vi "movement(a side) fwd use navX and Sonic.vi"(7 "angle Z(align)":ext, 8 "error in (no error)":errorcluster, 11 "distance":dbl) -> (0 "error out":errorcluster, 3 "angle Z":ext)   [LabVIEW 2017]
uses:
  <vilib>/myRIO/Common/Instrument Driver Framework/Utilities/typedefs/Generic FPGA Reference.ctl
  <vilib>/myRIO/Common/Instrument Driver Framework/Utilities/typedefs/myRIO v1.0 Reference.ctl
  <vilib>/myRIO/Common/Instrument Driver Framework/Utilities/typedefs/Hardware Version Enum.ctl
  <vilib>/myRIO/Common/Instrument Driver Framework/Utilities/typedefs/myRIO Generic Hardware Reference.ctl
  <vilib>/Instr/_visa.llb/VISA Configure Serial Port (Instr).vi
  <vilib>/userdefined/High Color/nirio_resource_hc.ctl
  <vilib>/myRIO/Common/Instrument Driver Framework/myRIO v1.0/Encoder/typedefs/Encoder Count Direction Enum.ctl
  <vilib>/myRIO/Common/Instrument Driver Framework/myRIO v1.0/Encoder/typedefs/Encoder Signal Mode.ctl
  <vilib>/myRIO/Common/Instrument Driver Framework/myRIO v1.0/Encoder/typedefs/Encoder Channels Enum.ctl
  <vilib>/myRIO/Instrument Drivers/Onboard IO/Encoder/typedefs/Encoder Reference.ctl
  <vilib>/myRIO/Instrument Drivers/Onboard IO/Encoder/Encoder.lvlib
  <vilib>/myRIO/Instrument Drivers/Onboard IO/Encoder/vis/Read.vi
  <vilib>/myRIO/Common/Instrument Driver Framework/myRIO v1.0/Encoder/typedefs/Encoder Configuration v1.0.ctl
  <vilib>/myRIO/Common/Instrument Driver Framework/myRIO v1.0/Encoder/vis/myRIO v1.1 Open Encoder.vi
  <vilib>/myRIO/Common/Instrument Driver Framework/myRIO v1.0/Encoder/vis/myRIO v1.0 Configure Encoder.vi
  <vilib>/myRIO/Instrument Drivers/Onboard IO/Encoder/vis/myRIO Encoder Open.xnode
  <vilib>/myRIO/Common/Instrument Driver Framework/Utilities/vis/Is FPGA Ref Available.vi
  <vilib>/myRIO/Express VI/Onboard IO/Encoder/Encoder Express VI.xnode
  <vilib>/myRIO/Instrument Drivers/Onboard IO/I2C/typedefs/I2C Transfer Rate.ctl
  <vilib>/myRIO/Instrument Drivers/Onboard IO/I2C/I2C.lvlib
  <vilib>/myRIO/Instrument Drivers/Onboard IO/I2C/typedefs/I2C Configuration.ctl
  <vilib>/myRIO/Common/Instrument Driver Framework/myRIO v1.0/I2C/typedefs/I2C Channels Enum.ctl
  <vilib>/myRIO/Instrument Drivers/Onboard IO/I2C/typedefs/I2C Reference.ctl
  <vilib>/myRIO/Instrument Drivers/Onboard IO/I2C/vis/myRIO I2C Open.xnode
  <vilib>/myRIO/Instrument Drivers/Utilities/Utilities.lvlib
  <vilib>/imath/engines/lvmath2/RunTimeEngine/Managers/WorkSpace/UID Generator.vi
  <vilib>/imath/engines/lvmath2/RunTimeEngine/LocalVariableDefStatement/MC_LocalVariableDefStatement_Display.vi
  <vilib>/imath/engines/lvmath2/RunTimeEngine/RunTimeType/NIMS_RunTimeType_From StrictType (excl LVString).vi
  <vilib>/imath/engines/lvmath2/RunTimeEngine/Managers/SymbolTable/Clear UID.vi
  <vilib>/imath/engines/lvmath2/RunTimeEngine/Managers/SymbolTable/NIMS_WorkSpace.lvlib
  <vilib>/imath/engines/lvmath2/RunTimeEngine/NodeEndStatement/NIMS_NodeEndStatement_Output.vi
  <vilib>/imath/engines/lvmath2/RunTimeEngine/ErrorHandling/NIMS_Finalize Error.vi
  <vilib>/imath/engines/lvmath2/RunTimeEngine/BuiltInFunctions/abs/NIMS_abs(signed).vi
  <vilib>/myRIO/Common/Instrument Driver Framework/myRIO v1.0/I2C/vis/myRIO v1.1 Open I2C.vi
panel:
  out "value Z":ext
  out "left_pwm":dbl
  out "right_pwm":dbl
  in  "stop":bool
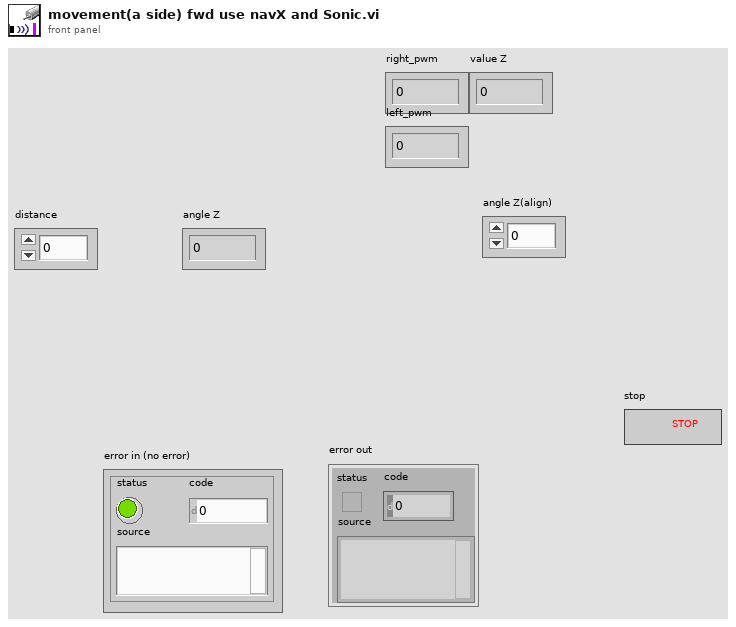
[diagram p1: front panel]
types:
  T1 = typedef "I2C.lvlib/I2C Reference.ctl" = cluster{"myRIO Reference":T2, "I2C Channels Enum":T6, "I2C Configuration":T7}
  T2 = typedef "myRIO Generic Hardware Reference.ctl" = cluster{"myRIO Model":T3, "myRIO Hardware Reference":T4}
  T3 = typedef "Hardware Version Enum.ctl" = enum16{"Unknown", "myRIO-1900", "myRIO-1950", "roboRIO", "NI ELVIS RIO CM"}
  T4 = typedef "myRIO v1.0 Reference.ctl" = cluster{"Generic FPGA Reference":T5, "Allow multiple opens":bool}
  T5 = typedef "Generic FPGA Reference.ctl" = refnum<k20>
  T6 = typedef "I2C Channels Enum.ctl" = enum16{"Not Connected", "A/I2C", "B/I2C", "I2C/I2C"}
  T7 = typedef "I2C.lvlib/I2C Configuration.ctl" = cluster{"I2C Transfer Rate":T8}
  T8 = typedef "I2C.lvlib/I2C Transfer Rate.ctl" = enum16{"Standard mode (100 kbps)", "Fast mode (400 kbps)"}
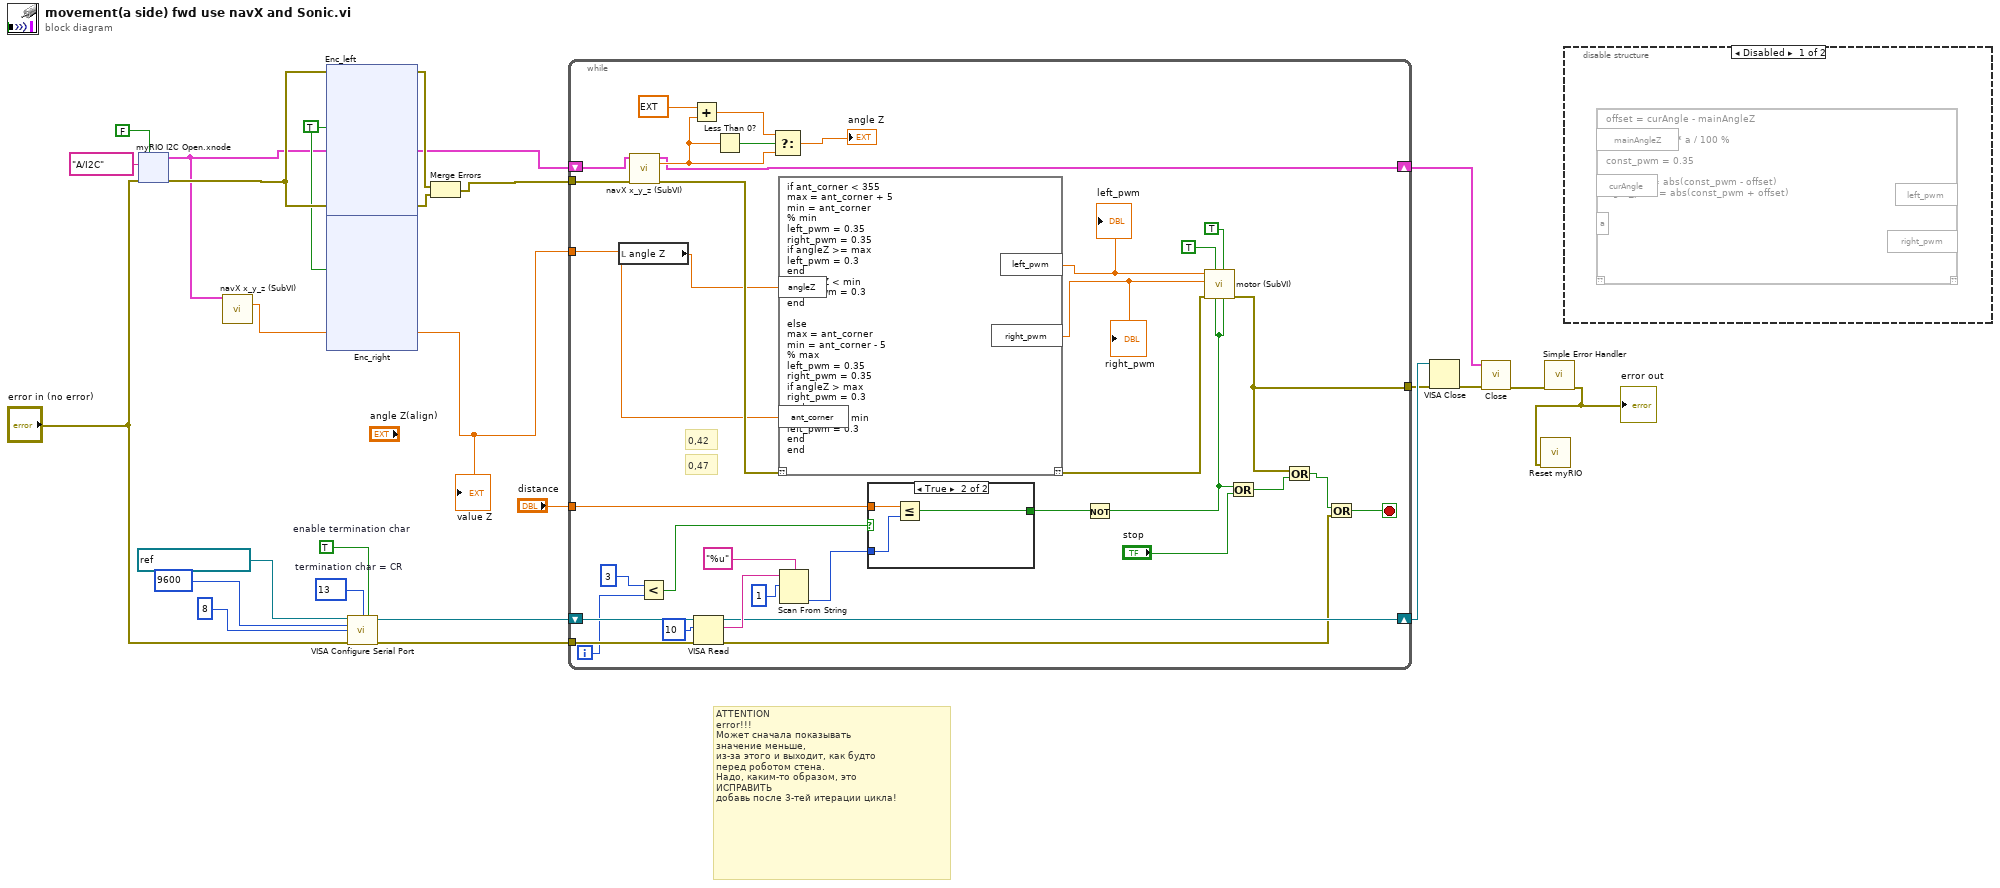
[diagram p0: block diagram]
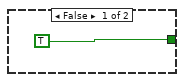
[diagram p3: hidden frame]
diagram:
  w5 = TRUE ("Reset Counter")
  w24 = u8 13  # termination char = CR
  w23 = TRUE  # enable termination char
  # "ATTENTION\nerror!!!\nМожет сначала показывать\nзначение меньше,\nиз-за этого и выходит, как будто \nперед роботом стена.\nНадо, каким-то образом, это\nИСПРАВИТЬ\nдобавь после 3-тей итерации цикла!"
  n1 = xnode "myRIO I2C Open.xnode"("error in (no error)"="error in (no error)", "Allow multiple opens?"=FALSE, "Channel Name"=tag "A/I2C") -> ("error out"=w14:errorcluster, "I2C Ref Out"=w2:T1)
  n2 = call "navX x_y_z (SubVI).vi"("I2C Ref Out in"=w2) -> ("value Z"=w1:ext)  [unwired: 10 in, 4 out]
  "value Z" <- w1
  n3 = xnode "Enc_left"("Reset Counter"=w5, "error in (no error)"=w14) -> ("error out"=w6:errorcluster)  [unwired: 3 out]
  n4 = xnode "Enc_right"("Reset Counter"=w5, "error in (no error)"=w14) -> ("error out"=w4:errorcluster)  [unwired: 3 out]
  n5 = call-poly "VISA Configure Serial Port"("VISA resource name"=refnum<visa-resource-name> "ASRL2::INSTR" ("UART selector"), "termination char\n(0xA = '\\n' = LF)"=w24, "Enable Termination\nChar (T)"=w23, "baud rate (9600)"=u32 9600 ("baud rate"), "data bits (8)"=u16 8 ("data bits"), "error in (no error)"="error in (no error)") -> ("VISA resource name out"=w18:refnum<visa-resource-name>, "error out"=w19:errorcluster)  [unwired: 8 in]
  n6 = Merge Errors(w6, w4) -> (w15:errorcluster)
  n7 = while {
    tunnel: w15 -> [w59]
    tunnel: w1 -> [w25]
    tunnel: [w51] -> w8
    tunnel: w19 -> [w44]
    tunnel: "distance" -> [w42]
    shift-right: [w46] -> w16
    shift-left: w18 -> [w45]
    shift-right: [w34] -> w10
    shift-left: w2 -> [w60]
    i -> [w37]
    stop <- w32 stop-if-true
    # "0,47"
    # "0,42"
    n8 = local read "angle Z"() -> (w26:ext)
    n9 = call "navX x_y_z (SubVI).vi"("I2C Ref Out in"=w60, "error in (no error)"=w59) -> ("I2C Ref Out out"=w34:T1, "value Z"=w54:ext, "error out"=w27:errorcluster)  [unwired: 9 in, 2 out]
    n10 = Less?(x=3, y=w37) -> (x < y?=w35:bool)
    n11 = Add(x=ext 360.0, y=w54) -> (x+y=w56:ext)
    n12 = VISA Read(VISA resource name=w45, byte count=u32 10, error in (no error)=w44) -> (VISA resource name out=w46:refnum<visa-resource-name>, read buffer=w47:string, error out=w31:errorcluster)  [unwired: 1 out]
    n13 = Less Than 0?(x=w54) -> (x < 0?=w58:bool)
    n14 = Select(t=w56, s=w58, f=w54) -> (s? t:f=→"angle Z":ext)
    n15 = mathscript code="if ant_corner < 355\nmax = ant_corner + 5\nmin = ant_corner\n% min\nleft_pwm = 0.35\nright_pwm = 0.35\nif angleZ >= max\nleft_pwm = 0.3\nend\nif angleZ < min\nright_pwm = 0.3\nend\n\nelse\nmax = ant_corner\nmin = ant_corner - 5\n% max\nleft_pwm = 0.35\nright_pwm = 0.35\nif angleZ > max\nright_pwm = 0.3\nend\nif angleZ <= min\nleft_pwm = 0.3\nend\nend"("??"=w27, "angleZ"=w26, "ant_corner"=w25) -> ("??"=w28:errorcluster, "right_pwm"=w29:dbl, "left_pwm"=w30:dbl)
    "right_pwm" <- w29
    "left_pwm" <- w30
    n16 = Scan From String(format string="%u", input string=w47, initial scan location=u32 1) -> (output 1=w43:u32)  [unwired: 2 in, 3 out]
    n17 = case shown="True" w35 {
      tunnel: w43 -> [_ w319]
      tunnel: w42 -> [_ w318]
      tunnel: [TRUE w317] -> w41
      frame False {
      }
      frame True {
        n18 = Less Or Equal?(x=w318, y=w319) -> (x <= y?=w317:bool)
      }
    }
    n19 = Not(x=w41) -> (.not. x?=w38:bool)
    n20 = call "motor (SubVI).vi"("M1 (Pin 26)"=w38, "M1 (Pin 25)"=TRUE, "M0 (Pin 23)"=w38, "M0 (Pin 21)"=TRUE, "error in (no error)"=w28, "PWM1"=w29, "PWM0"=w30) -> ("error out"=w51:errorcluster)  [unwired: 4 in]
    n21 = Or(x=w38, y="stop") -> (x .or. y?=w39:bool)
    n22 = Or(x=w51, y=w39) -> (x .or. y?=w33:bool)
    n23 = Or(x=w33, y=w31) -> (x .or. y?=w32:bool)
  }
  n24 = VISA Close(VISA resource name=w16, error in (no error)=w8) -> (error out=w7:errorcluster)
  n25 = call <vilib>:"Close.vi"("error in (no error)"=w7, "I2C Ref In"=w10) -> ("error out"=w9:errorcluster)  [unwired: 9 in]
  n26 = call <vilib>:"Simple Error Handler.vi"("error in (no error)"=w9) -> ("error out"=w3:errorcluster)  [unwired: 4 in, 4 out]
  "error out" <- w3
  n27 = call <vilib>:"Reset myRIO.vi"("error in (no error)"=w3) -> ()  [unwired: 10 in, 1 out]
  n28 = disable-structure shown="Disabled" {
    frame Disabled {
      n29 = mathscript code="offset = curAngle - mainAngleZ\n\noffset = offset * a / 100 %\n\nconst_pwm = 0.35\n\nleft_pwm = abs(const_pwm - offset)\nright_pwm = abs(const_pwm + offset)"() -> ()  [unwired: 4 in, 3 out]
    }
    frame Enabled {
    }
  }
